vi "CheckLightingConditions.vi"(4 "Bus Tape Gain":dbl=16.0, 5 "Change Lights? (Change; Coax; Spotlight)":bool[](array[boolean])=[FALSE, FALSE, FALSE], 6 "Si Gain":dbl, 8 "error in (no error)":errorcluster, 10 "Spotlights Refnum":refnum<vi>, 11 "Coaxial Lights Refnum":refnum<vi>) -> (0 "error out":errorcluster, 1 "Assigned Camera Gain":dbl, 2 "Spotlights Refnum out":refnum<vi>, 3 "Coaxial Lights Refnum out":refnum<vi>)   [LabVIEW 2017]
panel:
  out "Spotlights on?":bool
  out "Coaxial on?":bool
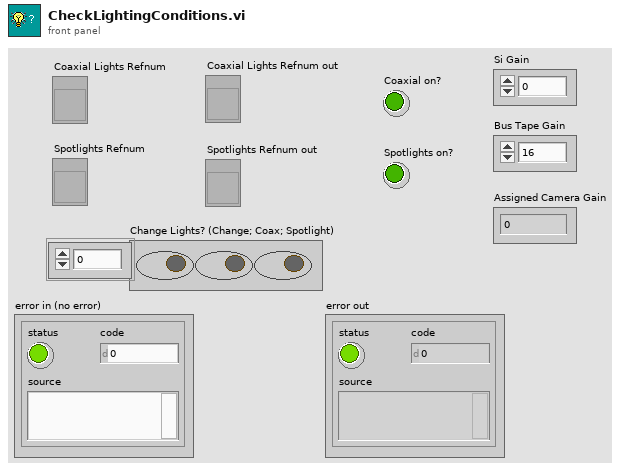
[diagram p1: front panel]
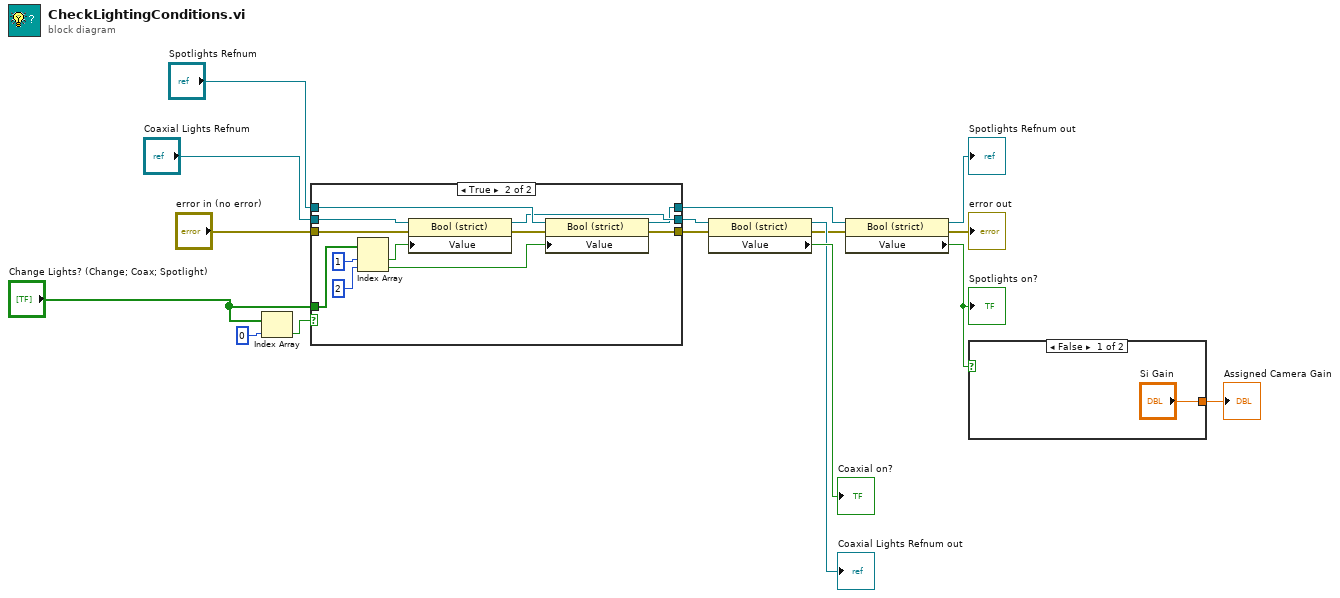
[diagram p0: block diagram]
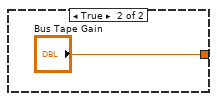
[diagram p3: hidden frame]
diagram:
  n1 = Index Array(array="Change Lights? (Change; Coax; Spotlight)", index=0) -> (element=w14:bool)
  n2 = case shown="True" w14 {
    tunnel: "Change Lights? (Change; Coax; Spotlight)" -> [_ w31]
    tunnel: "Coaxial Lights Refnum" -> [w19 w26]
    tunnel: "Spotlights Refnum" -> [w18 w25]
    tunnel: [w19 w24] -> w10
    tunnel: [w18 w23] -> w7
    tunnel: "error in (no error)" -> [w17 w22]
    tunnel: [w17 w20] -> w3
    frame False {
    }
    frame True {
      n3 = Index Array(array=w31, index #1=1 ("index"), index #2=2 ("index")) -> (element #1=w28:bool, element #2=w27:bool)
      n4 = property class="Bool (strict)"(reference=w26, error in=w22, "Value"=w28) -> (reference out=w24:refnum<vi>, error out=w21:errorcluster)
      n5 = property class="Bool (strict)"(reference=w25, error in=w21, "Value"=w27) -> (reference out=w23:refnum<vi>, error out=w20:errorcluster)
    }
  }
  n6 = property class="Bool (strict)"(reference=w10, error in=w3) -> (reference out=→"Coaxial Lights Refnum out":refnum<vi>, error out=w2:errorcluster, "Value"=→"Coaxial on?":bool)
  n7 = property class="Bool (strict)"(reference=w7, error in=w2) -> (reference out=→"Spotlights Refnum out":refnum<vi>, error out=→"error out":errorcluster, "Value"=w5:bool)
  "Spotlights on?" <- w5
  n8 = case shown="False" w5 {
    tunnel: ["Si Gain" "Bus Tape Gain"] -> w16
    frame False {
    }
    frame True {
    }
  }
  "Assigned Camera Gain" <- w16
